vi "Modify VI Icon Text Layer.vi"(8 "error in (no error)":errorcluster) -> (0 "error out":errorcluster)   [LabVIEW 2020, in "LabVIEW Icon API.lvlib"]
doc: "This example reads the current icon of a VI and updates it with an entirely new icon which primarily focuses on the Text Layer."
uses:
  <vilib>/LabVIEW Icon API/LabVIEW Icon API.lvlib
  <vilib>/Utility/miscctls.llb/LVRectTypeDef.ctl
panel:
  out "New VI Icon":picture
  out "Original VI Icon":picture
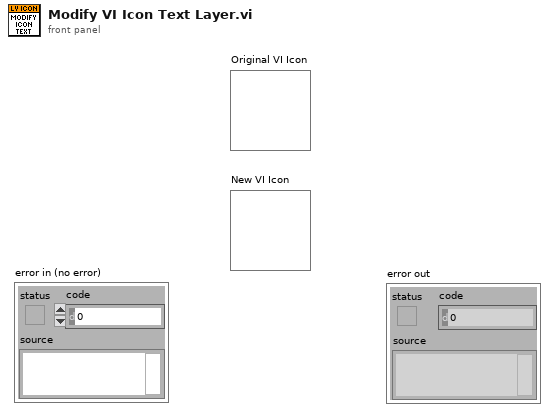
[diagram p1: front panel]
types:
  T1 = typedef "LVRectTypeDef.ctl" = cluster{"Left":i16, "Top":i16, "Right":i16, "Bottom":i16}
  T2 = typedef "imagedata.ctl" = cluster{"image type":i32, "image depth":i32, "image":u8[], "mask":u8[], "colors":u32[], "Rectangle":cluster{"left":i16, "top":i16, "right":i16, "bottom":i16}}
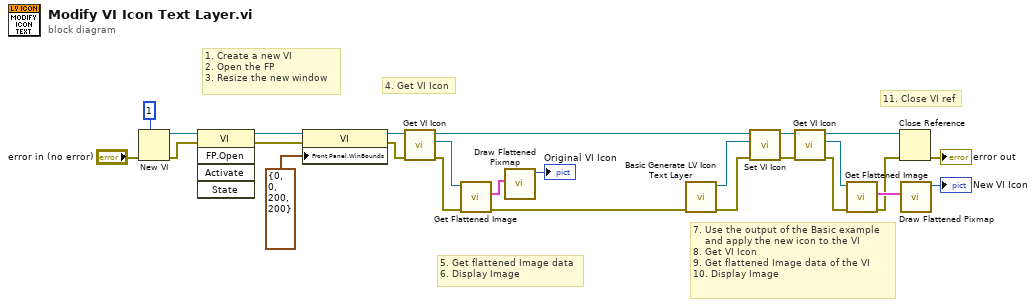
[diagram p0: block diagram]
diagram:
  # "11. Close VI ref"
  # "7. Use the output of the Basic example\n    and apply the new icon to the VI\n8. Get VI Icon\n9. Get flattened Image data of the VI\n10. Display Image"
  # "5. Get flattened Image data\n6. Display Image"
  # "4. Get VI Icon"
  # "1. Create a new VI\n2. Open the FP\n3. Resize the new window"
  n1 = New VI(7:u32 1 ("options"), 8:"error in (no error)") -> (0:w25:errorcluster, 3:w4:refnum<vi>)  [unwired: 5 in]
  n2 = invoke class="VI" method="FP.Open"(reference=w4, error in=w25) -> (reference out=w24:refnum<vi>, error out=w23:errorcluster)  [unwired: 3 in, 3 out]
  n3 = property class="VI"(reference=w24, error in=w23, "Front Panel.WinBounds"=T1 {"Left"=0, "Top"=0, "Right"=200, "Bottom"=200} ("Front Panel Window:Window Bounds")) -> (reference out=w21:refnum<vi>, error out=w20:errorcluster)
  n4 = call <vilib>:"Get VI Icon.vi"("error in (no error)"=w20, "VI Refnum in"=w21) -> ("error out"=w18:errorcluster, "Icon"=w19:refnum<class "Icon.lvclass">, "VI Refnum out"=w15:refnum<vi>)  [unwired: 7 in]
  n5 = call <vilib>:"Get Flattened Image.vi"("error in (no error)"=w18, "lv_icon.lvlib:Icon.lvclass in"=w19) -> ("error out"=w14:errorcluster, "Color Image"=w17:T2)  [unwired: 6 in, 2 out]
  n6 = call <vilib>:"Draw Flattened Pixmap.vi"("image data"=w17) -> ("new picture"=→"Original VI Icon":picture)  [unwired: 8 in]
  n7 = call <vilib>:"Basic Generate LV Icon Text Layer.vi"("error in (no error)"=w14) -> ("error out"=w13:errorcluster, "Icon.lvlclass out"=w12:refnum<class "Icon.lvclass">)  [unwired: 8 in, 1 out]
  n8 = call <vilib>:"Set VI Icon.vi"("error in (no error)"=w13, "Icon"=w12, "VI Refnum in"=w15) -> ("error out"=w9:errorcluster, "VI Refnum out"=w8:refnum<vi>)  [unwired: 7 in]
  n9 = call <vilib>:"Get VI Icon.vi"("error in (no error)"=w9, "VI Refnum in"=w8) -> ("error out"=w7:errorcluster, "Icon"=w6:refnum<class "Icon.lvclass">, "VI Refnum out"=w3:refnum<vi>)  [unwired: 7 in]
  n10 = call <vilib>:"Get Flattened Image.vi"("error in (no error)"=w7, "lv_icon.lvlib:Icon.lvclass in"=w6) -> ("error out"=w2:errorcluster, "Color Image"=w10:T2)  [unwired: 6 in, 2 out]
  n11 = Close Reference(reference=w3, error in (no error)=w2) -> (error out=→"error out":errorcluster)
  n12 = call <vilib>:"Draw Flattened Pixmap.vi"("image data"=w10) -> ("new picture"=→"New VI Icon":picture)  [unwired: 8 in]
